vi "Read True.vi"   [LabVIEW 2017, in "LabPack.lvlib" / "Reader.lvclass"]
uses:
  Reader.lvclass
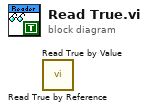
[diagram p0: block diagram]
diagram:
  n1 = call "Read True by Reference.vi"() -> ()  [unwired: 10 in, 2 out]
  n2 = call "Read True by Value.vi"() -> ()  [unwired: 10 in, 2 out]
